vi "Last_N_Samples_1D.vi"(1 "BufferLengthSamples":u32=100, 2 "InputArray":sgl[](array[numeric])) -> (0 "OutputArray":sgl[](array[numeric]))   [LabVIEW 2016]
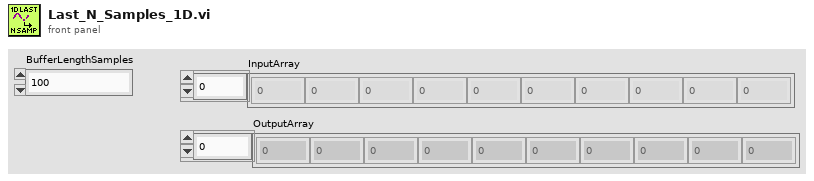
[diagram p1: front panel]
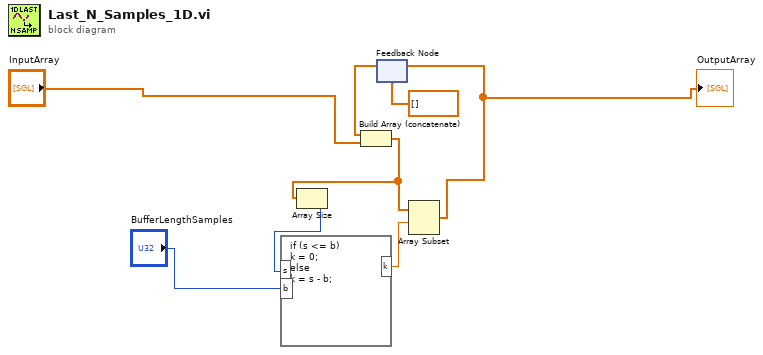
[diagram p0: block diagram]
diagram:
  n1 = feedback #1(sgl[] []) -> (w7:sgl[])
  n2 = Build Array (concatenate)(w7, "InputArray") -> (w6:sgl[])
  n3 = Array Size(array=w6) -> (size(s)=w5:i32)
  n4 = formula code="if (s <= b)\nk = 0;\nelse\nk = s - b;"("s"=w5, "b"="BufferLengthSamples") -> ("k"=w4:dbl)
  n5 = Array Subset(array=w6, index=w4) -> (w1:sgl[])  [unwired: 1 in]
  "OutputArray" <- w1
  n6 = feedback-in #1(w1) -> ()
